vi "AxisCardGlobal.vi"() -> ()   [LabVIEW 2019]
uses:
  AxisCard.lvclass
panel:
  out "CardClass":refnum<class "AxisCard.lvclass">[](array[class])
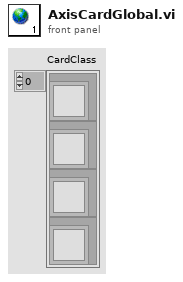
[diagram p1: front panel]
diagram:
